vi "1B_AnalyzePulseTrain_wOptions.vi"(0 "Waveform In":waveform(dbl)={"t0"=timestamp(3462203691.797 s since 1904-01-01), "dt"=1.428e-05, "Y"=array[8000 elements]}, 1 "Resampling Strength":T2, 5 "Repetitions in the Input Waveform":i32, 7 "Pulse Characteristics":T4={"Pulses per Cycle"=2, "Load Resistance (Ohms)"=750.0, "Krec Value"=2, "Recovery Mode (T=Active)"=TRUE, "Target Stim Currents (Amps)"=[]} {"Target Stim Currents (Amps)" format="%#.2p"}, 9 "Smoothing Strength":T3, 11 "Offset Calculation Method":T1=enum."Precise") -> (2 "Avg. CBC Width":dbl format="%0.6f", 3 "Avg. CBC Amplitude":dbl format="%0.2f", 4 "Stim PW":dbl[](array[numeric]) format="%#.3p", 6 "Stim Amplitude":dbl[](array[numeric]) format="%#.3p", 8 "Interphase Delay":dbl[](array[numeric]) format="%#.3p", 10 "Recovery PW":dbl[](array[numeric]) format="%#.3p", 12 "Waveform Parameters":T5 {"Frequency" format="%#.3p"; "Avg CBC Width" format="%.6f"; "Avg. CBC Holdoff" format="%#_6p"; "Stim Pulse Width" format="%#.3p"; "Interphase Delay" format="%#.3p"; "Recovery PW" format="%#_6p"; "Recovery Holdoff" format="%#.3p"; "Stim Amplitude" format="%#.3p"; "Recovery Amplitude" format="%#_6p"}, 13 "Frequency":dbl, 14 "Recovery Holdoff":dbl[](array[numeric]) format="%#.3p", 15 "Recovery Amplitude":dbl[](array[numeric]) format="%#.3p")   [LabVIEW 2010]
uses:
  FilterStrength.ctl
  1B_Resample Strength.ctl
  1B_Offset Calculation Method.ctl
panel:
  out "size":i32
  in  "View":enum32{"View All", "Graph Only"}(tab)
  out "Waveform in ( graph )":waveform(dbl)(graph)
  out "Normalized Waveform":waveform(dbl)(graph)
  out "(-) Offset":dbl
  out "Eq. Freq ( Hz )":dbl format="%#_6p"
  out "Current in amps":waveform(dbl)(graph)
  out "Time2 - Time1 ( sec )":dbl format="%#_6p"
  # "Tip: Select \"Simple\" if \"Precise\" cannot mesure offset"
  # "Remove idle voltage offset\n( if applicable )"
  # "The input waveform should be a capture of the STIM chip output\n(before the cap) when the output is held at 1/2 HVDD by the\nLoad Resistance.  This ensures that passive recovery and CBC\npulses are captured, because they look like pulses pulled to GND."
  # "The elements in these arrays correspond to the pulses per cycle.\nThey are the averages over all the repetitions in the waveform."
  # "Tip: Decreasing Repetitions may yield better results"
  # "Enter Target Current\nfor each in array below"
  # "1. Update Cursor Positions\n2. Turn off X Autoscaling\n3. Run this VI again"
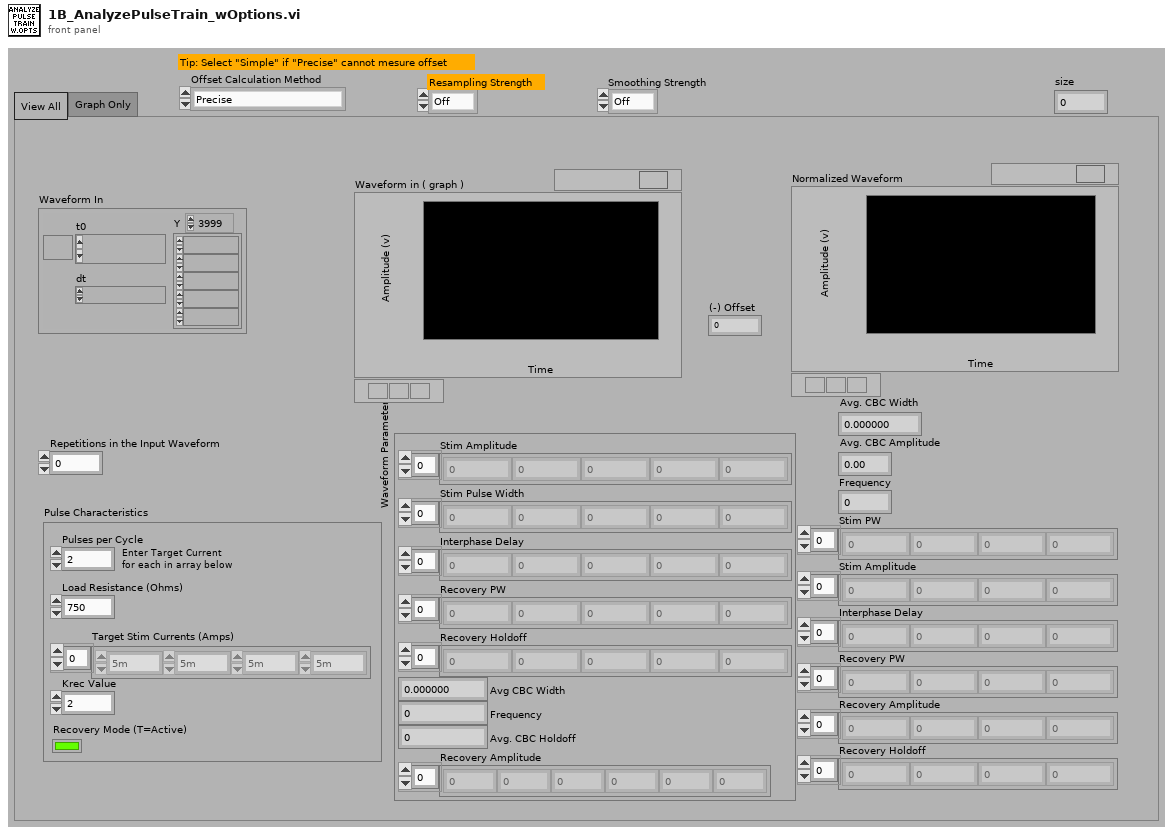
[diagram p1: front panel]
types:
  T1 = typedef "1B_Offset Calculation Method.ctl" = enum16{"Obsolete", "Precise", "Simple"}
  T2 = typedef "1B_Resample Strength.ctl" = enum16{"Off", "2", "4", "8", "16", "32"}
  T3 = typedef "FilterStrength.ctl" = enum16{"Off", "10", "20", "50", "100", "200", "500", "1000"}
  T4 = cluster{"Pulses per Cycle":i32, "Load Resistance (Ohms)":dbl, "Krec Value":i32, "Recovery Mode (T=Active)":bool, "Target Stim Currents (Amps)":dbl[]}
  T5 = cluster{"Stim Amplitude":dbl[], "Stim Pulse Width":dbl[], "Interphase Delay":dbl[], "Recovery PW":dbl[], "Recovery Holdoff":dbl[], "Avg CBC Width":dbl, "Frequency":dbl, "Avg. CBC Holdoff":dbl, "Recovery Amplitude":dbl[]}
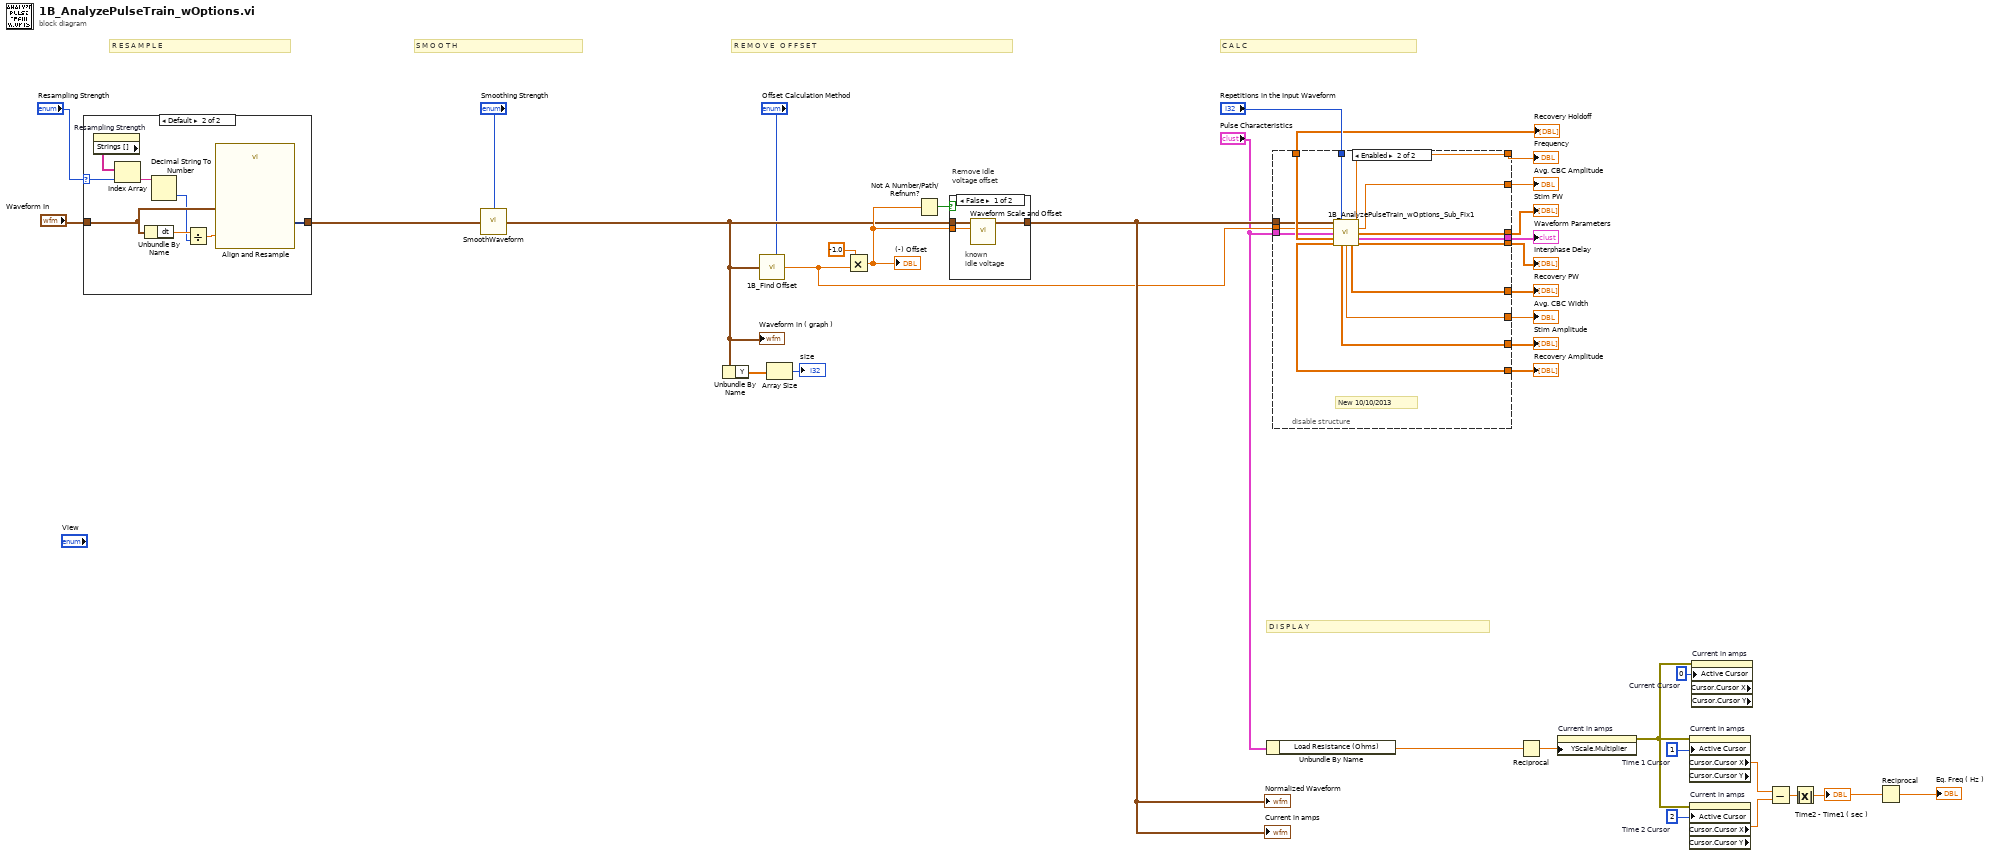
[diagram p0: block diagram]
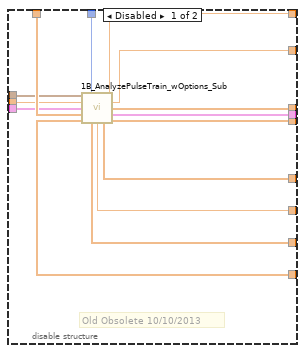
[diagram p2: hidden frame]
diagram:
  w13 = u32 0  # Current Cursor
  w20 = u32 2  # Time 2 Cursor
  w21 = u32 1  # Time 1 Cursor
  # "D I S P L A Y"
  # "C A L C"
  # "R E M O V E   O F F S E T"
  # "R E S A M P L E"
  # "S M O O T H"
  # "Remove idle voltage offset"
  n1 = case "R E S A M P L E" shown="Default" "Resampling Strength" {
    selector: "Resampling Strength" -> [_ w38]
    tunnel: "Waveform In" -> [w37 w42]
    tunnel: [w37 w43] -> w7
    frame "Off" {
    }
    frame Default {
      n2 = property on="Resampling Strength" class="Enum (strict)"() -> ("Strings []"=w40:string[])  [unwired: 2 in, 2 out]
      n3 = Index Array(array=w40, index=w38) -> (element=w41:string)
      n4 = Unbundle By Name(w42) -> ("dt"=w45:dbl)
      n5 = Decimal String To Number(string=w41) -> (number=w39:i32)  [unwired: 2 in, 1 out]
      n6 = Divide(x=w45, y=w39) -> (x/y=w44:dbl)
      n7 = call "Align and Resample"("dt"=w44, "Signals"=w42) -> ("Resampled Signals"=w43:dynamicdata)  [unwired: 7 in, 2 out]
    }
  }
  n8 = call "SmoothWaveform.vi"("Waveform"=w7, "Smoothing Strength"="Smoothing Strength") -> ("Filtered data"=w4:waveform(dbl))
  "Waveform in ( graph )" <- w4
  n9 = Unbundle By Name(w4) -> ("Y"=w6:dbl[])
  n10 = call "1B_Find Offset.vi"("Waveform"=w4, "Offset Calculation Method"="Offset Calculation Method") -> ("Offset"=w10:dbl)  [unwired: 1 in]
  n11 = Array Size(array=w6) -> (size(s)=→"size":i32)
  n12 = Multiply(x=-1.0, y=w10) -> (x*y=w24:dbl)
  "(-) Offset" <- w24
  n13 = Not A Number/Path/Refnum?(number/path/refnum=w24) -> (NaN/Path/Refnum?=w23:bool)
  n14 = case shown="False" w23 {
    tunnel: [w48 w49] -> w12
    tunnel: w4 -> [w47 w49]
    tunnel: w24 -> [w46 _]
    frame False {
      # "known\nidle voltage"
      n15 = call <vilib>:"Waveform Scale and Offset.vi"("offset"=w46, "waveform in"=w47) -> ("waveform out"=w48:waveform(dbl))  [unwired: 8 in, 1 out]
    }
    frame True {
      # "Unknown \nIdle Voltage"
    }
  }
  "Normalized Waveform" <- w12
  "Current in amps" <- w12
  n16 = Unbundle By Name("Pulse Characteristics") -> ("Load Resistance (Ohms)"=w1:dbl)
  n17 = disable-structure shown="Enabled" {
    disable-tunnel: "Repetitions in the Input Waveform" -> [w63 w77]
    disable-tunnel: [w62 w76] -> w34
    disable-tunnel: [w61 w75] -> w33
    disable-tunnel: [w60 w74] -> w32
    disable-tunnel: [w59 w73] -> w31
    disable-tunnel: [w58 w72] -> w30
    disable-tunnel: [w57 w71] -> w29
    disable-tunnel: [w56 w70] -> w28
    disable-tunnel: [w55 w69] -> w27
    disable-tunnel: [w54 w68] -> w26
    disable-tunnel: [w53 w67] -> w22
    disable-tunnel: w12 -> [w52 w66]
    disable-tunnel: w10 -> [w51 w65]
    disable-tunnel: "Pulse Characteristics" -> [w50 w64]
    frame Disabled {
      # "Old Obsolete 10/10/2013"
      n18 = call "1B_AnalyzePulseTrain_wOptions_Sub.vi"("Filtered data"=w52, "Repetitions in the Input Waveform"=w63, "Offset"=w51, "Pulse Characteristics"=w50) -> ("Frequency"=w62:dbl, "Avg. CBC Amplitude"=w61:dbl, "Stim PW"=w60:dbl[], "Recovery Holdoff"=w55:dbl[], "Waveform Parameters"=w53:T5, "Recovery Amplitude"=w56:dbl[], "Stim Amplitude"=w57:dbl[], "Avg. CBC Width"=w54:dbl, "Recovery PW"=w58:dbl[], "Interphase Delay"=w59:dbl[])  [unwired: 2 in]
    }
    frame Enabled {
      # "New 10/10/2013"
      n19 = call "1B_AnalyzePulseTrain_wOptions_Sub_Fix1.vi"("Filtered data"=w66, "Repetitions in the Input Waveform"=w77, "Offset"=w65, "Pulse Characteristics"=w64) -> ("Frequency"=w76:dbl, "Avg. CBC Amplitude"=w75:dbl, "Stim PW"=w74:dbl[], "Recovery Holdoff"=w69:dbl[], "Waveform Parameters"=w67:T5, "Recovery Amplitude"=w70:dbl[], "Stim Amplitude"=w71:dbl[], "Avg. CBC Width"=w68:dbl, "Recovery PW"=w72:dbl[], "Interphase Delay"=w73:dbl[])  [unwired: 2 in]
    }
  }
  "Stim PW" <- w32
  "Interphase Delay" <- w31
  "Recovery PW" <- w30
  "Recovery Holdoff" <- w27
  "Stim Amplitude" <- w29
  "Recovery Amplitude" <- w28
  "Avg. CBC Width" <- w26
  "Avg. CBC Amplitude" <- w33
  "Frequency" <- w34
  "Waveform Parameters" <- w22
  n20 = Reciprocal(x=w1) -> (1/x=w25:dbl)
  n21 = property on="Current in amps" class="WFGraph (strict)"("YScale.Multiplier"=w25) -> (error out=w14:errorcluster)  [unwired: 2 in, 1 out]
  n22 = property on="Current in amps" class="WFGraph (strict)" props=["Active Cursor", "Cursor", "Cursor X", "Cursor", "Cursor Y"](error in=w14, "Active Cursor"=w21) -> ("Cursor.Cursor X"=w18:dbl)  [unwired: 1 in, 3 out]
  n23 = property on="Current in amps" class="WFGraph (strict)" props=["Active Cursor", "Cursor", "Cursor X", "Cursor", "Cursor Y"](error in=w14, "Active Cursor"=w20) -> ("Cursor.Cursor X"=w17:dbl)  [unwired: 1 in, 3 out]
  n24 = property on="Current in amps" class="WFGraph (strict)" props=["Active Cursor", "Cursor", "Cursor X", "Cursor", "Cursor Y"](error in=w14, "Active Cursor"=w13) -> ()  [unwired: 1 in, 4 out]
  n25 = Subtract(x=w18, y=w17) -> (x-y=w19:dbl)
  n26 = Absolute Value(x=w19) -> (abs(x)=w16:dbl)
  "Time2 - Time1 ( sec )" <- w16
  n27 = Reciprocal(x=w16) -> (1/x=→"Eq. Freq ( Hz )":dbl)
